vi "TestDatabaseControllerGFV.vi"   [LabVIEW 2017]
uses:
  DatabaseContollerGFVenum.ctl
types:
  T1 = typedef "DatabaseContollerGFVenum.ctl" = enum16{"Init and Open Database!", "Close Database!", "Get Users!"}
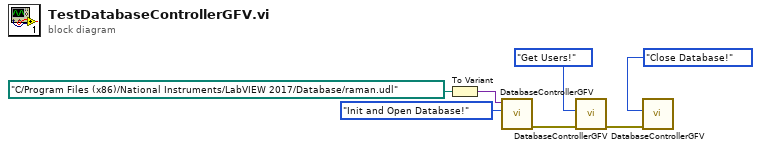
[diagram p0: block diagram]
diagram:
  n1 = To Variant(anything=path "C:/Program Files (x86)/National Instruments/LabVIEW 2017/Database/raman.udl" ("connection information")) -> (Variant=w6:variant)
  n2 = call "DatabaseControllerGFV.vi"("Enum"=DatabaseContollerGFVenum."Init and Open Database!", "Data in"=w6) -> ("error out"=w4:errorcluster)  [unwired: 8 in, 1 out]
  n3 = call "DatabaseControllerGFV.vi"("error in (no error)"=w4, "Enum"=DatabaseContollerGFVenum."Get Users!") -> ("error out"=w2:errorcluster)  [unwired: 8 in, 1 out]
  n4 = call "DatabaseControllerGFV.vi"("error in (no error)"=w2, "Enum"=DatabaseContollerGFVenum."Close Database!") -> ()  [unwired: 8 in, 2 out]
